vi "Convert Params to String.vi"(11 "Settings":T1={"Step Values"=[], "Only Execute When Test Running"=FALSE, "Reset Sequence When Test Starts"=TRUE, "Current Sequence ID"=0, "Total Iterations"=0, "Current Step Start Timestamp"=0.0, "Number of Sequence Steps"=0, "Num of Analog Channels"=0, "Num of Digital Channels"=0, "Delay Before Starting Sequence"=0.0, "Show UI"=FALSE, "Time Remaining"=0.0, "Test Running"=FALSE, "Pause Timestamp"=0.0}) -> (3 "String out":string)   [LabVIEW 2024, in "Sequencer with Output Values.lvlib" / "Sequencer with Output Values.lvclass"]
uses:
  Sequencer with Output Values.lvclass
  Params.ctl
  Step Settings.ctl
  Global Strings.vi
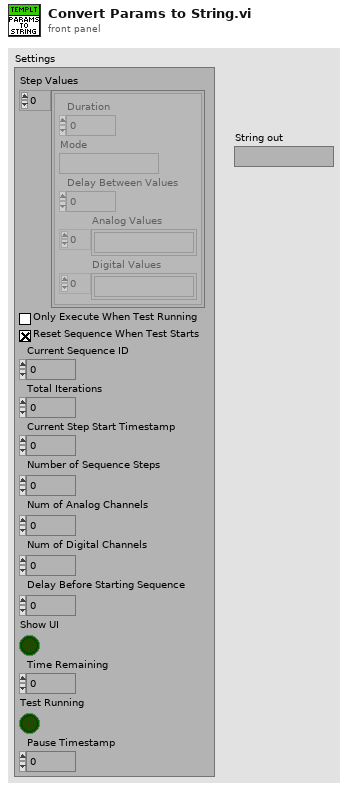
[diagram p1: front panel]
types:
  T1 = typedef "Sequencer with Output Values.lvlib/Sequencer with Output Values.lvclass/Params.ctl" = cluster{"Step Values":T2[], "Only Execute When Test Running":bool, "Reset Sequence When Test Starts":bool, "Current Sequence ID":u32, "Total Iterations":u32, "Current Step Start Timestamp":dbl, "Number of Sequence Steps":i32, "Num of Analog Channels":i32, "Num of Digital Channels":i32, "Delay Before Starting Sequence":dbl, "Show UI":bool, "Time Remaining":dbl, "Test Running":bool, "Pause Timestamp":dbl}
  T2 = typedef "Sequencer with Output Values.lvlib/Sequencer with Output Values.lvclass/Step Settings.ctl" = cluster{"Duration":dbl, "Mode":string, "Delay Between Values":dbl, "Analog Values":string[], "Digital Values":string[]}
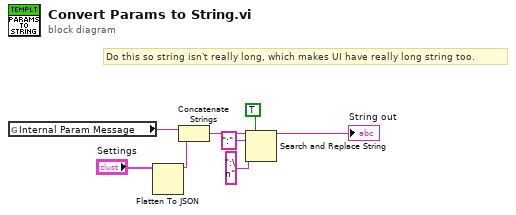
[diagram p0: block diagram]
diagram:
  # "Do this so string isn't really long, which makes UI have really long string too."
  n1 = global read "Global Strings.vi" "Internal Param Message"() -> (w1:string)
  n2 = Flatten To JSON(anything="Settings") -> (JSON string=w3:string)  [unwired: 2 in, 1 out]
  n3 = Concatenate Strings(w1, w3) -> (w7:string)
  n4 = Search and Replace String(replace all?=TRUE ("replace all? (F)"), input string=w7, search string=":", replace string=":\n" ("replace string (\"\")")) -> (result string=→"String out":string)  [unwired: 4 in, 3 out]
